vi "APS get error position.vi"(8 "error in (no error)":errorcluster caption="错误输入（无错误）", 10 "Err_Pos":i32, 11 "Axis_ID":i32) -> (0 "error out":errorcluster caption="错误输出", 2 "Err_Pos out":i32, 3 "function return":i32)   [LabVIEW 2012, in "APS168.lvlib"]
doc: "I32 FNTYPE APS_get_error_position( I32 Axis_ID, I32 *Err_Pos );"
uses:
  APS168.lvlib
  APS168.dll
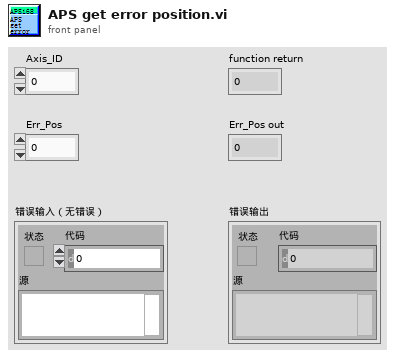
[diagram p1: front panel]
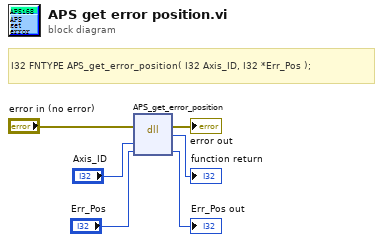
[diagram p0: block diagram]
diagram:
  # "I32 FNTYPE APS_get_error_position( I32 Axis_ID, I32 *Err_Pos );"
  n1 = dll-call lib="PTH1/abs E\t冲压机LLB运动204cAPS168.*" fn="APS_get_error_position"(error in="error in (no error)", "Axis_ID"="Axis_ID", "Err_Pos"="Err_Pos") -> (error out=→"error out":errorcluster, →"function return":i32, "Err_Pos"=→"Err_Pos out":i32)  [unwired: 3 in, 1 out]
